vi "MB Ethernet Receive.vi"(8 "error in (no error)":errorcluster, 9 "Timeout":i32=5000, 11 "Connection ID":refnum<k5>) -> (0 "error out":errorcluster, 1 "Exception Code":u8 format="%.0x", 2 "Modbus Data Unit":T2={"Function Code"=1, "Data"=[]} {"Function Code" items=["Read Coils"=1, "Read Discrete Inputs"=2, "Read Holding Registers"=3, "Read Input Registers"=4, "Write Single Coil"=5, "Write Single Register"=6, "Read Exception Status"=7, "Write Multiple Coils"=15, "Write Multiple Registers"=16]; "Data" format="%.0x"}, 3 "Connection ID (dup)":refnum<k5>, 5 "MBAP Header":T1)   [LabVIEW 2011]
uses:
  MB Modbus Data Unit.ctl
panel:
  # "VI Name: MB Ethernet Receive.vi\nPurpose: Reads a Modbus message over Ethernet.\nReentrant VI, because its caller is also reentrant."
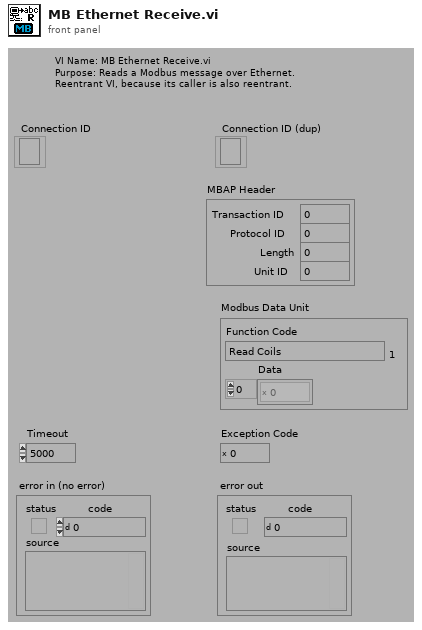
[diagram p1: front panel]
types:
  T1 = cluster{"Transaction ID":u16, "Protocol ID":u16, "Length":u16, "Unit ID":u8}
  T2 = typedef "MB Modbus Data Unit.ctl" = cluster{"Function Code":u8, "Data":u8[]}
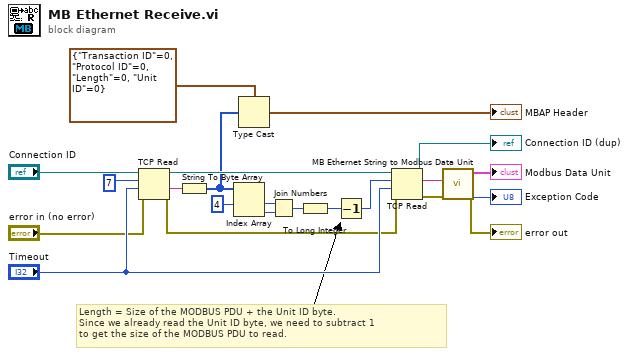
[diagram p0: block diagram]
diagram:
  # "Length = Size of the MODBUS PDU + the Unit ID byte.\nSince we already read the Unit ID byte, we need to subtract 1\nto get the size of the MODBUS PDU to read."
  n1 = TCP Read(connection ID="Connection ID", bytes to read=7, error in (no error)="error in (no error)", 9:"Timeout") -> (connection ID out=w20:refnum<k5>, data out=w19:string, error out=w13:errorcluster)  [unwired: 1 out]
  n2 = String To Byte Array(string=w19) -> (unsigned byte array=w9:u8[])
  n3 = Index Array(array=w9, index #1=4 ("index")) -> (element #1=w14:u8, element #2=w15:u8)  [unwired: 1 in]
  n4 = Type Cast(type=T1 {"Transaction ID"=0, "Protocol ID"=0, "Length"=0, "Unit ID"=0} ("MBAP Header"), x=w9) -> (*(type *) &x=→"MBAP Header":T1)
  n5 = Join Numbers(hi=w14, lo=w15) -> ((hi.lo)=w17:u16)
  n6 = To Long Integer(number=w17) -> (32bit integer=w16:i32)
  n7 = Decrement(x=w16) -> (x-1=w12:i32)
  n8 = TCP Read(connection ID=w20, bytes to read=w12, error in (no error)=w13, 9:"Timeout") -> (connection ID out=→"Connection ID (dup)":refnum<k5>, data out=w10:string, error out=w5:errorcluster)  [unwired: 1 out]
  n9 = call "MB Ethernet String to Modbus Data Unit.vi"("error in (no error)"=w5, "String"=w10) -> ("error out"=→"error out":errorcluster, "Exception Code"=→"Exception Code":u8, "Modbus Data Unit"=→"Modbus Data Unit":T2)  [unwired: 7 out]
